vi "Create Image Overlay with Pupil Center.vi"(10 "Circles":T1(array[cluster]), 11 "Refnum in":T2) -> (3 "Refnum out":T2)   [LabVIEW 2015]
uses:
  <vilib>/vision/Image Controls.llb/IMAQ Image.ctl
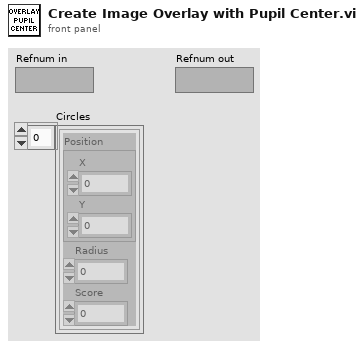
[diagram p1: front panel]
types:
  T1 = cluster{"Position":cluster{"X":sgl, "Y":sgl}, "Radius":dbl, "Score":dbl}[]
  T2 = typedef "IMAQ Image.ctl" = refnum<image>
  T3 = cluster{"Left":i32, "Top":i32, "Right":i32, "Bottom":i32}
  T4 = cluster{"Position":cluster{"X":sgl, "Y":sgl}, "Radius":dbl, "Score":dbl}
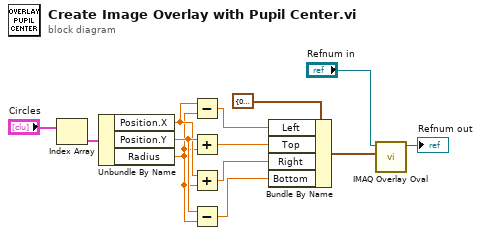
[diagram p0: block diagram]
diagram:
  n1 = Index Array(array="Circles") -> (element=w4:T4)  [unwired: 1 in]
  n2 = Unbundle By Name(w4) -> ("Position.X"=w2:sgl, "Position.Y"=w3:sgl, "Radius"=w1:dbl)
  n3 = Subtract(x=w2, y=w1) -> (x-y=w9:dbl)
  n4 = Add(x=w3, y=w1) -> (x+y=w6:dbl)
  n5 = Add(x=w2, y=w1) -> (x+y=w8:dbl)
  n6 = Subtract(x=w3, y=w1) -> (x-y=w7:dbl)
  n7 = Bundle By Name(cluster=T3 {"Left"=0, "Top"=0, "Right"=0, "Bottom"=0} ("Bounding Rectangle"), "Left"=w9, "Top"=w6, "Right"=w8, "Bottom"=w7) -> (w5:T3)
  n8 = call "IMAQ Overlay Oval"("Bounding Rectangle"=w5, "Image"="Refnum in") -> ("Image Out"=→"Refnum out":T2)  [unwired: 8 in, 1 out]
